vi "rotate 2d array up.vi"(10 "From Facet":i32[][](array[numeric])=[[3, 4, 5], [1, 4, 7], [3, 4, 8], [7, 4, 1]], 11 "Ring":T1 items=["Up"=-1, "Down"=1]) -> (2 "Rotated":i32[][](array[numeric]), 3 "Dup Original":i32[][](array[numeric])=[[3, 4, 5], [1, 4, 7], [3, 4, 8], [7, 4, 1]])   [LabVIEW 2019]
uses:
  Rotate array command.ctl
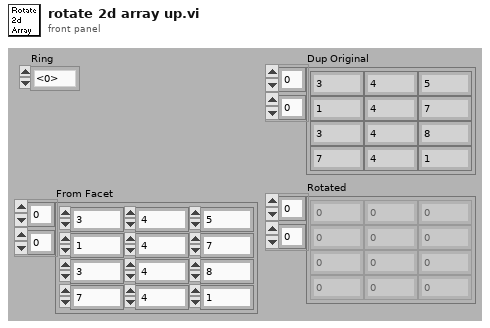
[diagram p1: front panel]
types:
  T1 = typedef "Rotate array command.ctl" = i32
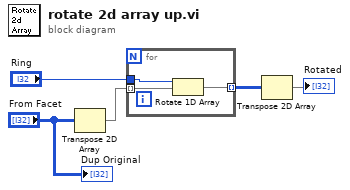
[diagram p0: block diagram]
diagram:
  n1 = Transpose 2D Array(2D array="From Facet") -> (transposed array=w4:i32[][])
  n2 = for {
    tunnel: w4 -> [w8] mode=indexing
    tunnel: [w7] -> w3 mode=indexing
    tunnel: "Ring" -> [w6]
    n3 = Rotate 1D Array(1:w8, 2:w6) -> (0:w7:i32[])
  }
  n4 = Transpose 2D Array(2D array=w3) -> (transposed array=→"Rotated":i32[][])
  "Dup Original" <- "From Facet"
